vi "Get.vi"(8 "error in (no error)":errorcluster, 11 "queue":refnum<queue>) -> (0 "error out":errorcluster, 1 "Data":variant, 2 "Command":string, 3 "queue out":refnum<queue>, 4 "timed out?":bool)   [LabVIEW 2016, in "System Queue.lvlib"]
uses:
  System Queue.lvlib
  Control_Queue Data.ctl
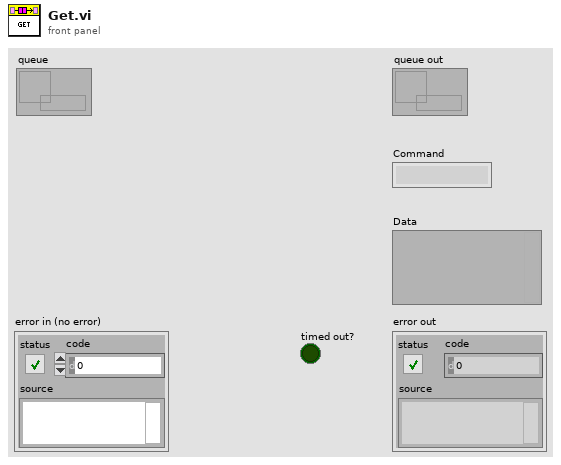
[diagram p1: front panel]
types:
  T1 = typedef "System Queue.lvlib/Control_Queue Data.ctl" = cluster{"Command":string, "Data":variant}
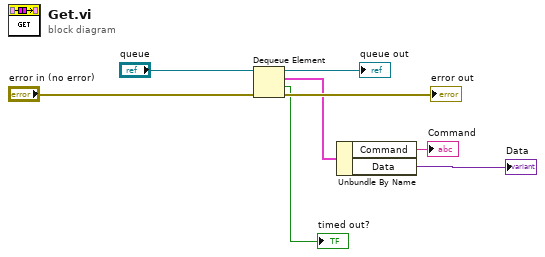
[diagram p0: block diagram]
diagram:
  n1 = Dequeue Element(queue="queue", error in (no error)="error in (no error)") -> (queue out=→"queue out":refnum<queue>, element=w3:T1, timed out?=→"timed out?":bool, error out=→"error out":errorcluster)  [unwired: 1 in]
  n2 = Unbundle By Name(w3) -> ("Command"=→"Command":string, "Data"=→"Data":variant)
